vi "Post-Build Action.vi"(4 "measurement plugin service":refnum<class "Measurement Plugin Service.lvclass">, 5 "files generated by build":path[](array[path]), 6 "top level/always included VIs":path[](array[path]), 7 "destination path":path, 8 "error in":errorcluster, 9 "target name":string, 10 "build specification name":string, 11 "project path":path) -> (0 "error out":errorcluster)   [LabVIEW 2020, in "MeasurementLink Measurement Server.lvlib"]
uses:
  MeasurementLink Measurement Server.lvlib
  <vilib>/Utility/config.llb/NI_LVConfig.lvlib
  <vilib>/ErrorRing/Error Ring.xnode
  Measurement Plugin Service/Measurement Plugin Service.lvclass
  <vilib>/Utility/config.llb/Write Key (String).vi
  User Interface Type.ctl
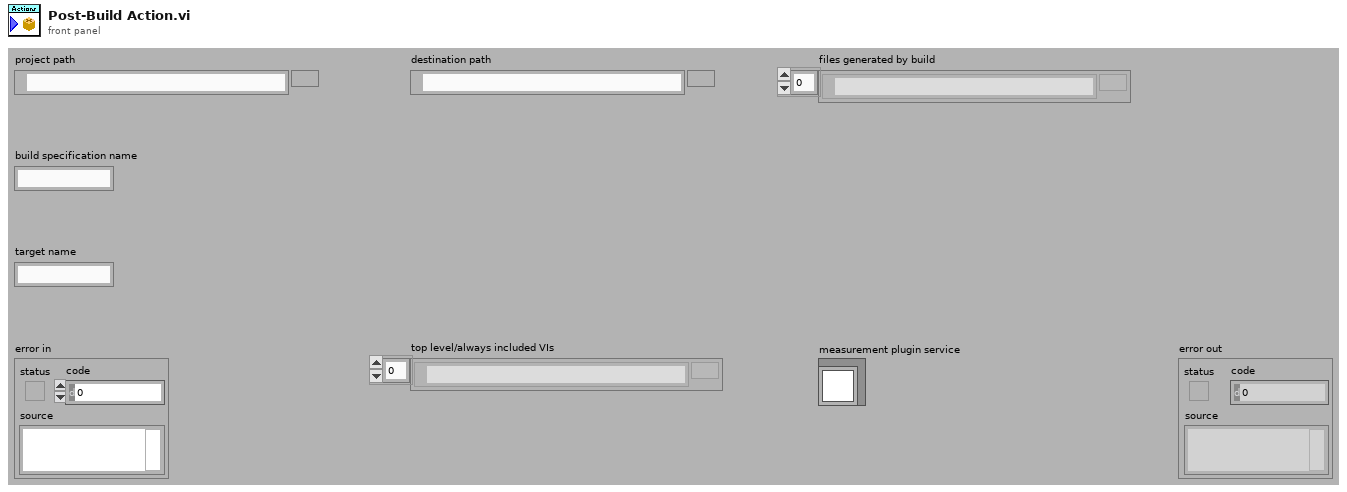
[diagram p1: front panel]
types:
  T1 = cluster{"target name":string, "top level/always included VIs":path[], "project path":path, "destination path":path, "build specification name":string, "files generated by build":path[]}
  T2 = typedef "MeasurementLink Measurement Server.lvlib/User Interface Type.ctl" = enum16{"Loose VI", "VI in lvlib", "VI in lvlibp"}
  T3 = typedef "MeasurementLink Measurement Server.lvlib/User Interface Details.ctl" = cluster{"file url":string}
  T4 = typedef "MeasurementLink Measurement Server.lvlib/Measurement Details.ctl" = cluster{"display name":string, "version":string}
  T5 = typedef "MeasurementLink Measurement Server.lvlib/Measurement Annotation.ctl" = cluster{"key":string, "value":string}
  T6 = typedef "NI_LVConfig.lvlib/Config Data RefNum.ctl" = refnum<k1>
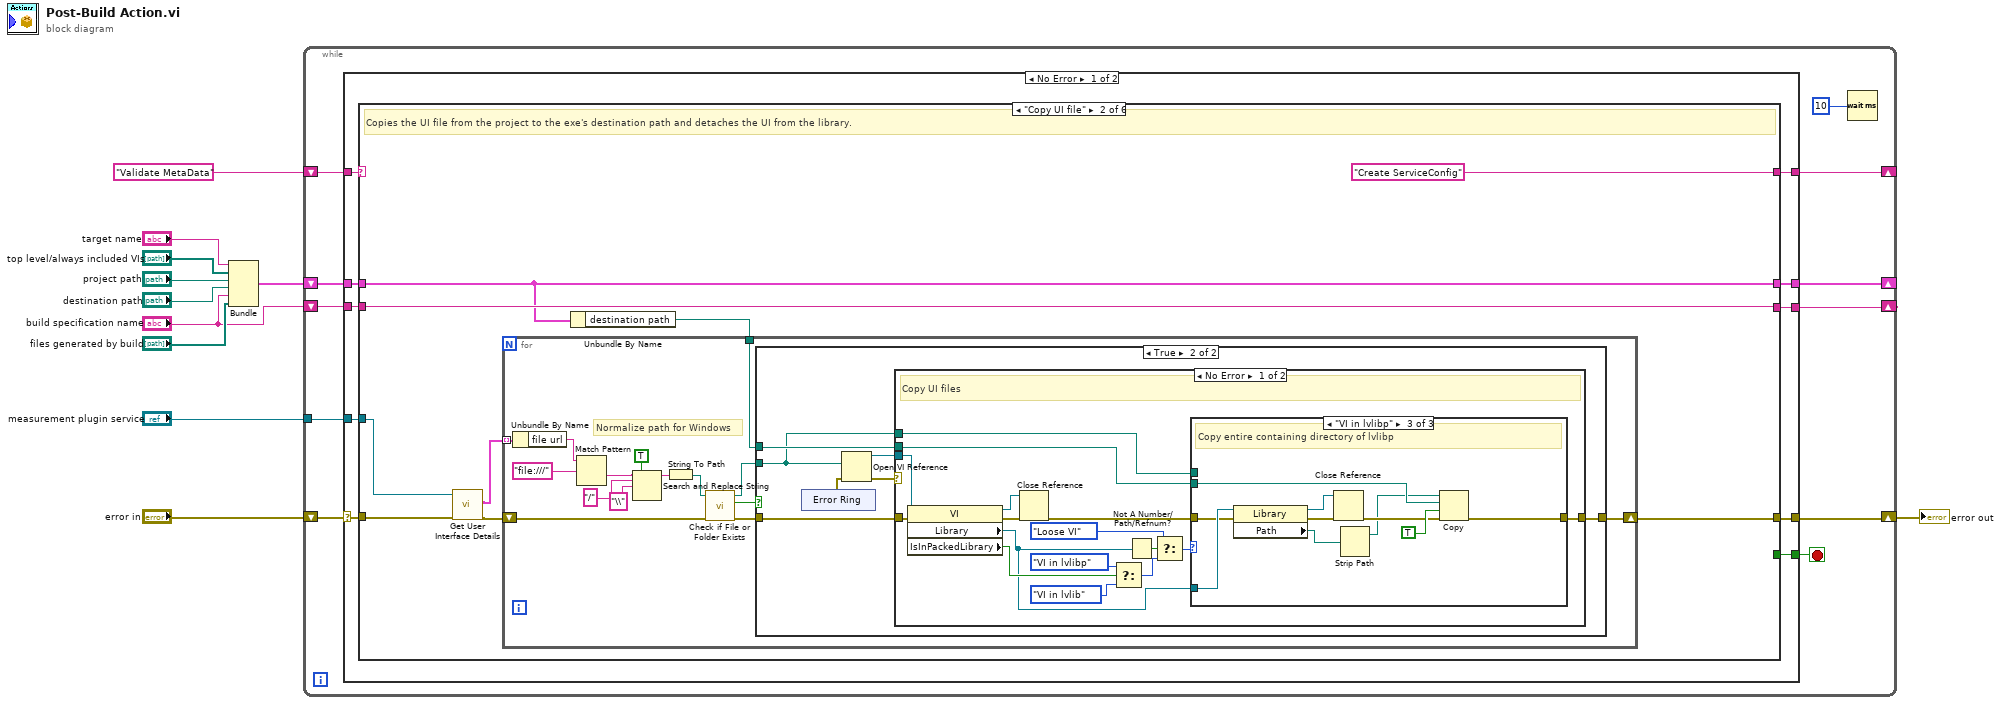
[diagram p0: block diagram]
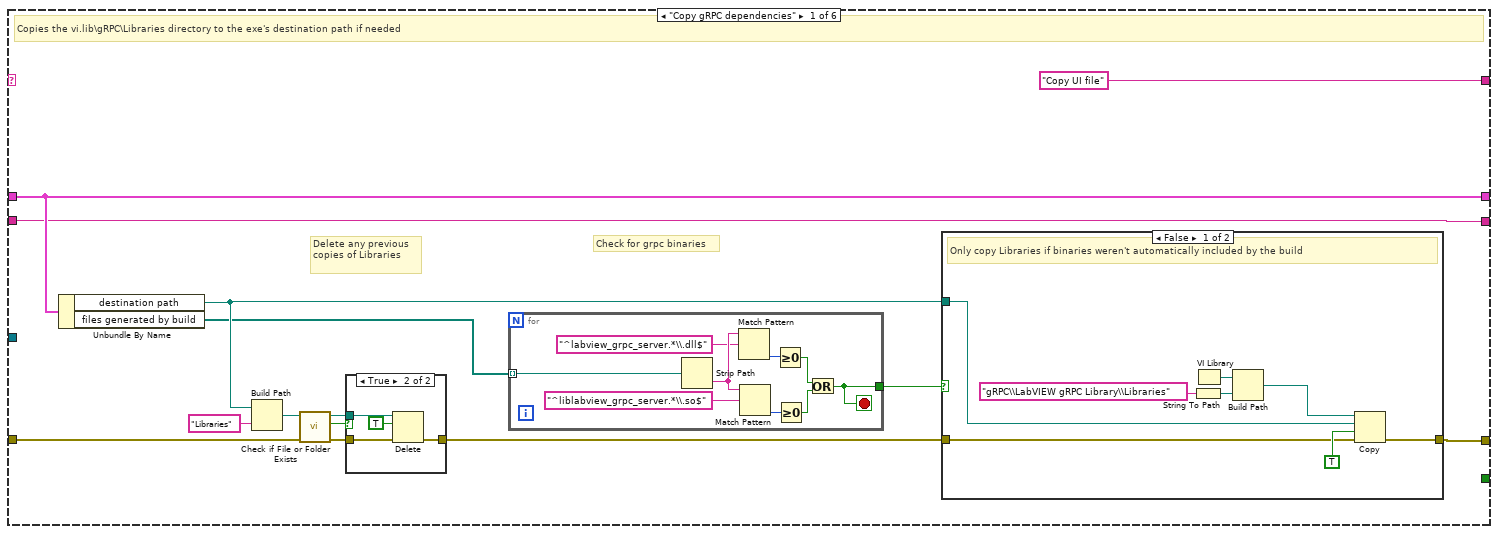
[diagram p2: hidden frame]
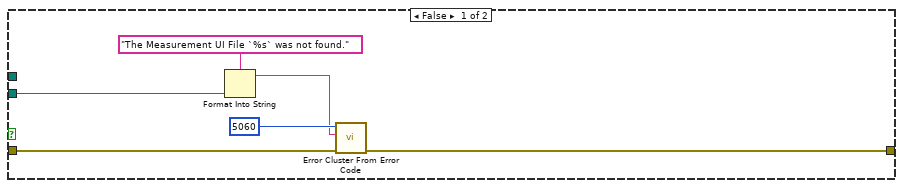
[diagram p5: hidden frame]
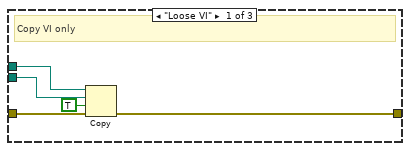
[diagram p6: hidden frame]
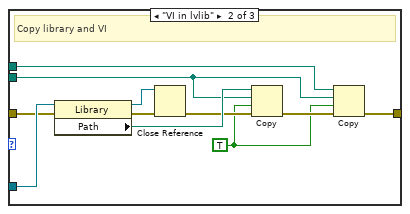
[diagram p7: hidden frame]
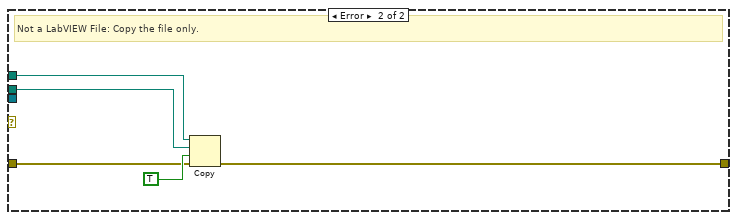
[diagram p8: hidden frame]
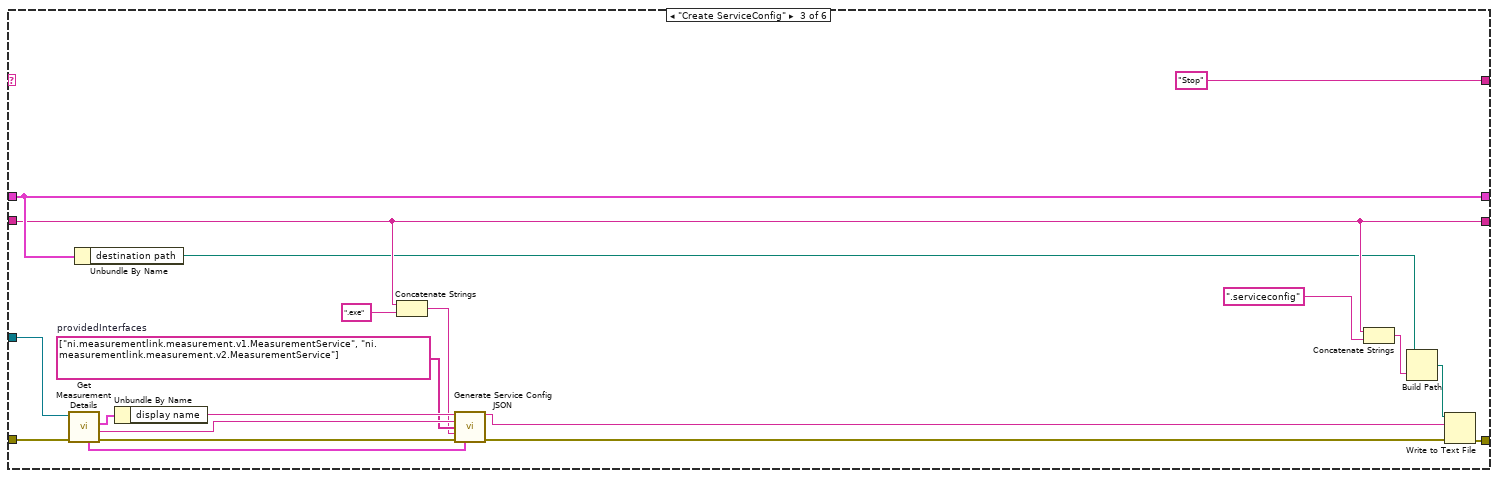
[diagram p9: hidden frame]
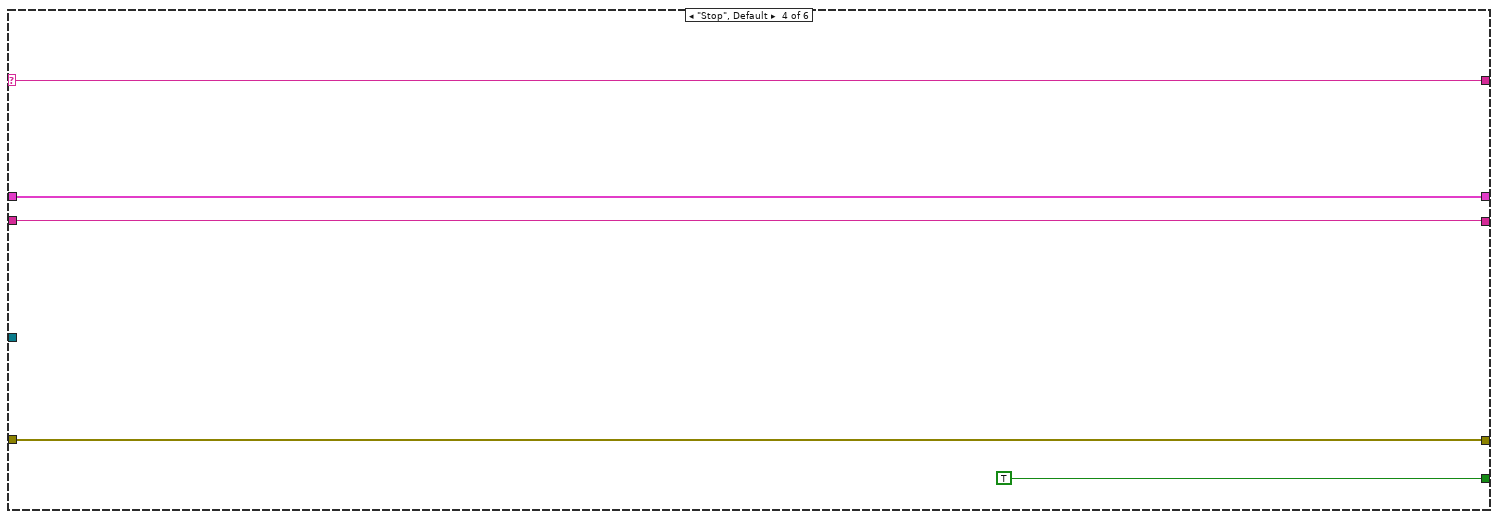
[diagram p10: hidden frame]
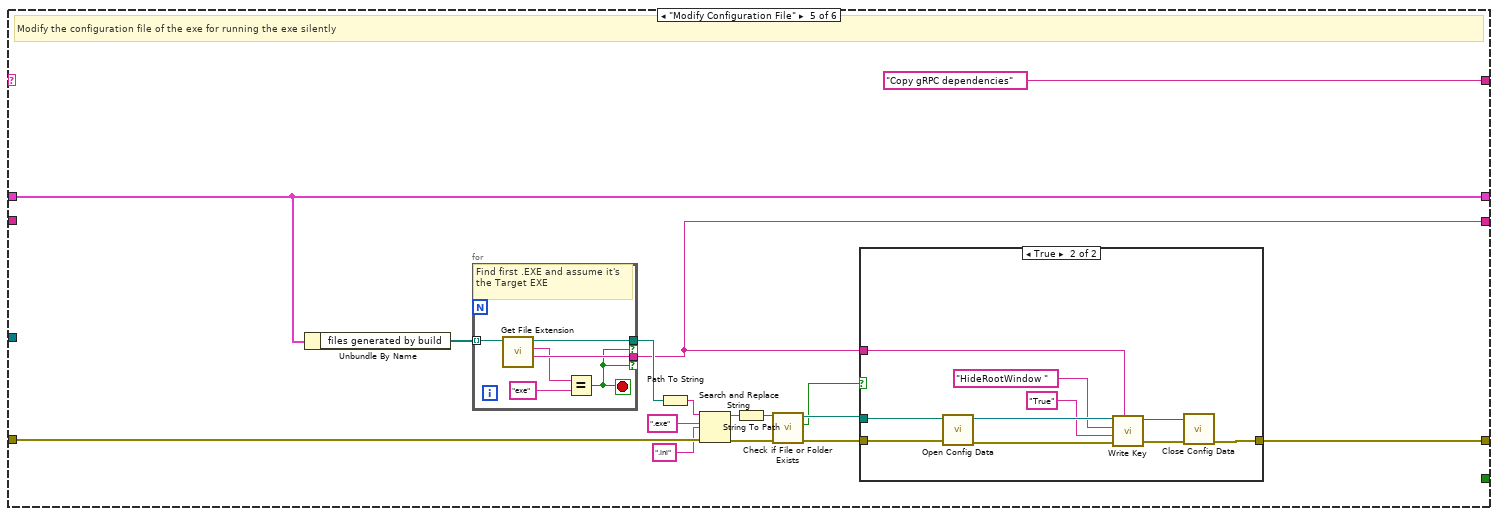
[diagram p11: hidden frame]
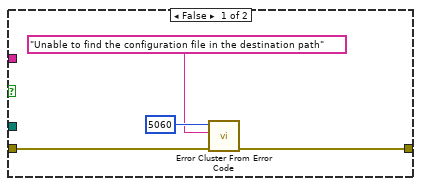
[diagram p12: hidden frame]
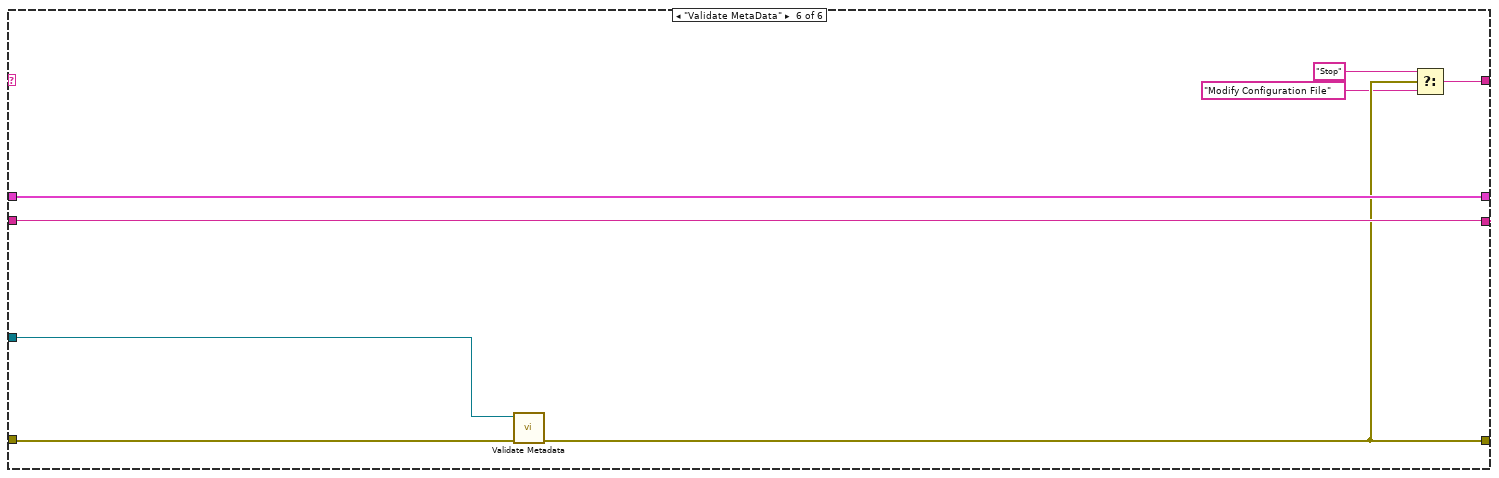
[diagram p13: hidden frame]
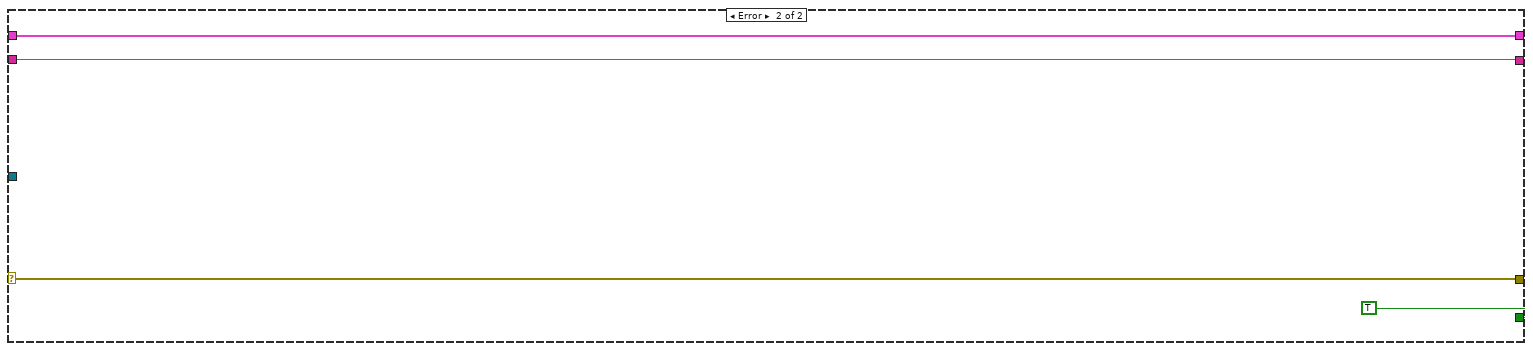
[diagram p14: hidden frame]
diagram:
  n1 = Bundle("target name"="target name", "top level/always included VIs"="top level/always included VIs", "project path"="project path", "destination path"="destination path", "build specification name"="build specification name", "files generated by build"="files generated by build") -> (w5:T1)  [unwired: 1 in]
  n2 = while {
    shift-right: [w19] -> _
    shift-left: w5 -> [w20]
    shift-right: [w18] -> w3
    shift-left: "error in" -> [w15]
    shift-right: [w17] -> _
    shift-left: "Validate MetaData" -> [w21]
    shift-right: [w14] -> _
    shift-left: "build specification name" -> [w13]
    tunnel: "measurement plugin service" -> [w12]
    stop <- w16 stop-if-true
    n3 = case shown="No Error" w15 {
      selector: w15 -> [w26 w226]
      tunnel: w21 -> [w32 _]
      tunnel: w20 -> [w31 w227]
      tunnel: [w30 w227] -> w19
      tunnel: [w29 w226] -> w18
      tunnel: [w28 _] -> w17
      tunnel: [w27 TRUE] -> w16
      tunnel: [w25 w224] -> w14
      tunnel: w13 -> [w24 w224]
      tunnel: w12 -> [w23 _]
      frame No Error {
        n4 = case shown="\"Copy UI file\"" w32 {
          selector: w32 -> [_ _ _ w177 _ _]
          tunnel: w31 -> [w44 w75 w174 w179 w191 w223]
          tunnel: [w44 w75 w174 w179 w191 w223] -> w30
          tunnel: w26 -> [w36 w73 w164 w176 w189 w221]
          tunnel: [w46 w74 w167 w176 w195 w219] -> w29
          tunnel: ["Copy UI file" "Create ServiceConfig" "Stop" w177 "Copy gRPC dependencies" w216] -> w28
          tunnel: [_ _ _ TRUE _ _] -> w27
          tunnel: [w43 w77 w171 w175 w181 w222] -> w25
          tunnel: w24 -> [w43 w77 w171 w175 _ w222]
          tunnel: w23 -> [_ w71 w165 _ _ w220]
          frame "Copy gRPC dependencies" {
            # "Delete any previous copies of Libraries"
            # "Check for grpc binaries"
            # "Copies the vi.lib\\gRPC\\Libraries directory to the exe's destination path if needed"
            n5 = Unbundle By Name(w44) -> ("destination path"=w35:path, "files generated by build"=w33:path[])
            n6 = Build Path(base path=w35, name or relative path="Libraries") -> (appended path=w41:path)
            n7 = call <vilib>:"Check if File or Folder Exists.vi"("error in (no error)"=w36, "path"=w41) -> ("error out"=w40:errorcluster, "file or folder exists?"=w38:bool, "dup path"=w39:path)  [unwired: 7 in]
            n8 = case shown="True" w38 {
              tunnel: w40 -> [w56 w60]
              tunnel: [w56 w59] -> w34
              tunnel: w39 -> [_ w57]
              frame False {
              }
              frame True {
                n9 = Delete(path (use dialog)=w57, entire hierarchy (F)=TRUE ("confirm (F)"), error in=w60) -> (error out=w59:errorcluster)  [unwired: 2 in, 2 out]
              }
            }
            n10 = for {
              tunnel: [w47] -> w42
              tunnel: w33 -> [w52] mode=indexing
              stop <- w47 stop-if-true
              n11 = Strip Path(path=w52) -> (name=w55:string)  [unwired: 1 out]
              n12 = Match Pattern(string=w55, regular expression="^labview_grpc_server.*\\.dll$" ("pattern")) -> (offset past match=w51:i32)  [unwired: 1 in, 3 out]
              n13 = Match Pattern(string=w55, regular expression="^liblabview_grpc_server.*\\.so$" ("pattern")) -> (offset past match=w50:i32)  [unwired: 1 in, 3 out]
              n14 = Greater Or Equal To 0?(x=w51) -> (x >= 0?=w49:bool)
              n15 = Greater Or Equal To 0?(x=w50) -> (x >= 0?=w48:bool)
              n16 = Or(x=w49, y=w48) -> (x .or. y?=w47:bool)
            }
            n17 = case shown="False" w42 {
              tunnel: [w64 w69] -> w46
              tunnel: w35 -> [w62 _]
              tunnel: w34 -> [w61 w69]
              frame False {
                # "Only copy Libraries if binaries weren't automatically included by the build"
                n18 = String To Path(string="gRPC\\LabVIEW gRPC Library\\Libraries") -> (path=w66:path)
                n19 = VI Library() -> (path=w68:path)
                n20 = Build Path(base path=w68, name or relative path=w66) -> (appended path=w65:path)
                n21 = Copy(8:w61, 9:TRUE ("overwrite (F)"), 10:w62, 11:w65) -> (0:w64:errorcluster)  [unwired: 1 in, 2 out]
              }
              frame True {
              }
            }
          }
          frame "Copy UI file" {
            # "Copies the UI file from the project to the exe's destination path and detaches the UI from the library."
            n22 = call-dynamic "Get User Interface Details.vi"("error in"=w73, "measurement plugin service in"=w71) -> ("error out"=w72:errorcluster, "user interface details"=w70:T3[])  [unwired: 7 in, 1 out]
            n23 = Unbundle By Name(w75) -> ("destination path"=w76:path)
            n24 = for {
              tunnel: w76 -> [w89]
              tunnel: w70 -> [w92] mode=indexing
              shift-right: [w93] -> w74
              shift-left: w72 -> [w88]
              # "Normalize path for Windows"
              n25 = Unbundle By Name(w92) -> ("file url"=w90:string)
              n26 = Match Pattern(string=w90, regular expression="file:///") -> (after substring=w83:string)  [unwired: 1 in, 3 out]
              n27 = Search and Replace String(replace all?=TRUE ("replace all? (F)"), input string=w83, search string="/" ("after substring"), replace string="\\" ("after substring")) -> (result string=w82:string)  [unwired: 4 in, 3 out]
              n28 = String To Path(string=w82) -> (path=w86:path)
              n29 = call <vilib>:"Check if File or Folder Exists.vi"("error in (no error)"=w88, "path"=w86) -> ("error out"=w87:errorcluster, "file or folder exists?"=w84:bool, "dup path"=w85:path)  [unwired: 7 in]
              n30 = case shown="True" w84 {
                tunnel: [w97 w106] -> w93
                tunnel: w89 -> [_ w102]
                tunnel: w87 -> [w98 w101]
                tunnel: w85 -> [w95 w100]
                frame False {
                  n31 = Format Into String(format string="The Measurement UI File `%s` was not found." ("error message (\"\")"), w95) -> (resulting string=w94:string)  [unwired: 2 in, 1 out]
                  n32 = call <vilib>:"Error Cluster From Error Code.vi"("error in (no error)"=w98, "error message (\"\")"=w94, "error code (0)"=5060) -> ("error out"=w97:errorcluster)  [unwired: 6 in]
                }
                frame True {
                  n33 = xnode "Error Ring"() -> ("error out"=w105:errorcluster)
                  n34 = Open VI Reference(vi path=w100, error in (no error)=w105) -> (vi reference=w103:refnum<vi>, error out=w104:errorcluster)  [unwired: 4 in]
                  n35 = case shown="No Error" w104 {
                    tunnel: w101 -> [w122 w153]
                    tunnel: [w120 w152] -> w106
                    tunnel: w103 -> [w123 _]
                    tunnel: w102 -> [w119 w151]
                    tunnel: w100 -> [w118 w150]
                    frame No Error {
                      # "Copy UI files"
                      n36 = property class="VI"(reference=w123, error in=w122) -> (reference out=w116:refnum<vi>, error out=w121:errorcluster, "Library"=w108:refnum<vi>, "IsInPackedLibrary"=w113:bool)
                      n37 = Close Reference(reference=w116, error in (no error)=w121) -> (error out=w117:errorcluster)
                      n38 = Select(t=User_Interface_Type."VI in lvlibp", s=w113, f=User_Interface_Type."VI in lvlib") -> (s? t:f=w110:T2)
                      n39 = Not A Number/Path/Refnum?(number/path/refnum=w108) -> (NaN/Path/Refnum?=w115:bool)
                      n40 = Select(t=User_Interface_Type."Loose VI", s=w115, f=w110) -> (s? t:f=w109:T2)
                      n41 = case shown="\"VI in lvlibp\"" w109 {
                        tunnel: [w124 w132 w142] -> w120
                        tunnel: w108 -> [_ w139 w149]
                        tunnel: w117 -> [w128 w138 w148]
                        tunnel: w119 -> [w127 w130 w143]
                        tunnel: w118 -> [w126 w131 _]
                        frame "Loose VI" {
                          # "Copy VI only"
                          n42 = Copy(8:w128, 9:TRUE ("overwrite (F)"), 10:w127, 11:w126) -> (0:w124:errorcluster)  [unwired: 1 in, 2 out]
                        }
                        frame "VI in lvlib" {
                          w129 = TRUE ("overwrite (F)")
                          # "Copy library and VI"
                          n43 = property class="Library"(reference=w139, error in=w138) -> (reference out=w134:refnum<vi>, error out=w136:errorcluster, "Path"=w137:path)
                          n44 = Close Reference(reference=w134, error in (no error)=w136) -> (error out=w135:errorcluster)
                          n45 = Copy(8:w135, 9:w129, 10:w130, 11:w137) -> (0:w133:errorcluster)  [unwired: 1 in, 2 out]
                          n46 = Copy(8:w133, 9:w129, 10:w130, 11:w131) -> (0:w132:errorcluster)  [unwired: 1 in, 2 out]
                        }
                        frame "VI in lvlibp" {
                          # "Copy entire containing directory of lvlibp"
                          n47 = property class="Library"(reference=w149, error in=w148) -> (reference out=w144:refnum<vi>, error out=w146:errorcluster, "Path"=w141:path)
                          n48 = Close Reference(reference=w144, error in (no error)=w146) -> (error out=w145:errorcluster)
                          n49 = Strip Path(path=w141) -> (stripped path=w140:path)  [unwired: 1 out]
                          n50 = Copy(8:w145, 9:TRUE ("overwrite (F)"), 10:w143, 11:w140) -> (0:w142:errorcluster)  [unwired: 1 in, 2 out]
                        }
                      }
                    }
                    frame Error {
                      # "Not a LabVIEW File: Copy the file only."
                      n51 = Copy(8:w153, 9:TRUE ("overwrite (F)"), 10:w151, 11:w150) -> (0:w152:errorcluster)  [unwired: 1 in, 2 out]
                    }
                  }
                }
              }
            }
          }
          frame "Create ServiceConfig" {
            w159 = string[] ["ni.measurementlink.measurement.v1.MeasurementService", "ni.measurementlink.measurement.v2.MeasurementService"]  # providedInterfaces
            n52 = call-dynamic "Get Measurement Details.vi"("error in"=w164, "measurement plugin service in"=w165) -> ("error out"=w162:errorcluster, "service class"=w160:string, "measurement details"=w163:T4, "measurement annotations"=w157:T5[])  [unwired: 5 in, 1 out]
            n53 = Unbundle By Name(w174) -> ("destination path"=w169:path)
            n54 = Unbundle By Name(w163) -> ("display name"=w161:string)
            n55 = Concatenate Strings(w171, ".exe" ("string")) -> (w158:string)
            n56 = call "Generate Service Config JSON.vi"("display name"=w161, "service class"=w160, "provided interfaces"=w159, "path"=w158, "error in"=w162, "annotations"=w157) -> ("service config JSON"=w155:string, "error out"=w156:errorcluster)  [unwired: 8 in]
            n57 = Concatenate Strings(w171, ".serviceconfig" ("string")) -> (w168:string)
            n58 = Build Path(base path=w169, name or relative path=w168) -> (appended path=w166:path)
            n59 = Write to Text File(file (use dialog)=w166, text=w155, error in=w156) -> (error out=w167:errorcluster)  [unwired: 1 in, 2 out]
          }
          frame "Stop", Default {
          }
          frame "Modify Configuration File" {
            # "Modify the configuration file of the exe for running the exe silently"
            n60 = Unbundle By Name(w191) -> ("files generated by build"=w190:path[])
            n61 = for {
              tunnel: w190 -> [w201] mode=indexing
              tunnel: [w200] -> w181 if=w196
              tunnel: [w199] -> w183 if=w196
              stop <- w196 stop-if-true
              # "Find first .EXE and assume it's the Target EXE"
              n62 = call <vilib>:"Get File Extension.vi"("file"=w201) -> ("filename without extension"=w200:string, "lowercase file extension"=w197:string, "dup file"=w199:path)  [unwired: 6 in, 2 out]
              n63 = Equal?(x=w197, y="exe") -> (x = y?=w196:bool)
            }
            n64 = Path To String(path=w183) -> (string=w182:string)
            n65 = Search and Replace String(input string=w182, search string=".exe", replace string=".ini", error in=w189) -> (result string=w186:string, error out=w188:errorcluster)  [unwired: 4 in, 2 out]
            n66 = String To Path(string=w186) -> (path=w185:path)
            n67 = call <vilib>:"Check if File or Folder Exists.vi"("error in (no error)"=w188, "path"=w185) -> ("error out"=w194:errorcluster, "file or folder exists?"=w192:bool, "dup path"=w193:path)  [unwired: 7 in]
            n68 = case shown="True" w192 {
              tunnel: [w204 w215] -> w195
              tunnel: w193 -> [_ w208]
              tunnel: w194 -> [w205 w207]
              tunnel: w181 -> [_ w206]
              frame False {
                n69 = call <vilib>:"Error Cluster From Error Code.vi"("error in (no error)"=w205, "error message (\"\")"="Unable to find the configuration file in the destination path" ("source"), "error code (0)"=5060) -> ("error out"=w204:errorcluster)  [unwired: 6 in]
              }
              frame True {
                n70 = call <vilib>:"Open Config Data.vi"("error in (no error)"=w207, "configuration file path"=w208) -> ("error out"=w214:errorcluster, "refnum"=w213:T6)  [unwired: 7 in, 1 out]
                n71 = call-poly <vilib>:"Write Key.vi"("section"=w206, "error in (no error)"=w214, "value"="True", "key"="HideRootWindow ", "refnum"=w213) -> ("error out"=w211:errorcluster, "refnum out"=w210:T6)  [unwired: 4 in, 1 out]
                n72 = call <vilib>:"Close Config Data.vi"("error in (no error)"=w211, "refnum"=w210) -> ("error out"=w215:errorcluster)  [unwired: 8 in, 1 out]
              }
            }
          }
          frame "Validate MetaData" {
            n73 = call "Validate Metadata.vi"("error in"=w221, "measurement plugin service in"=w220) -> ("error out"=w219:errorcluster)  [unwired: 8 in, 1 out]
            n74 = Select(t="Stop", s=w219, f="Modify Configuration File") -> (s? t:f=w216:string)
          }
        }
      }
      frame Error {
      }
    }
    n75 = Wait (ms)(milliseconds to wait=u32 10 ("millisecond timer value")) -> ()  [unwired: 1 out]
  }
  "error out" <- w3
